vi "SSL Data Receiver.vi"(11 "SSL Data 2":refnum<vi>) -> (2 "SSL RefBox":T1, 3 "SSL Vision":T1)   [LabVIEW 2017]
uses:
  <extravilib>/ChannelInstances/Lossy Stream-a[.](u8)/)Channel.ctl
  Control/SSL Data Control.ctl
  Control/SSL UDP Address.ctl
  Control/File Player.ctl
  <extravilib>/ChannelInstances/Lossy Stream-a[.](u8)/Write With Abort.vi
  <extravilib>/ChannelInstances/Lossy Stream-a[.](u8)/Endpoint.vi
  <extravilib>/ChannelInstances/Stream-a[.](u8)/Instantiate.vi
  <extravilib>/ChannelInstances/Lossy Stream-a[.](u8)/Instantiate.vi
  <extravilib>/ChannelInstances/Lossy Stream-a[.](u8)/)Channel.vi
  <extravilib>/ChannelInstances/Lossy Stream-a[.](u8).lvlib
panel:
  in  "Boolean 2":refnum<vi>
  in  "Cluster in":refnum<vi>
  in  "RefBox UDP RX":refnum<vi>
  in  "SSL UDP RX":refnum<vi>
  out "error out":errorcluster
  out "error out 4":errorcluster
  out "error out":errorcluster
  # "UDP"
  # "LOG"
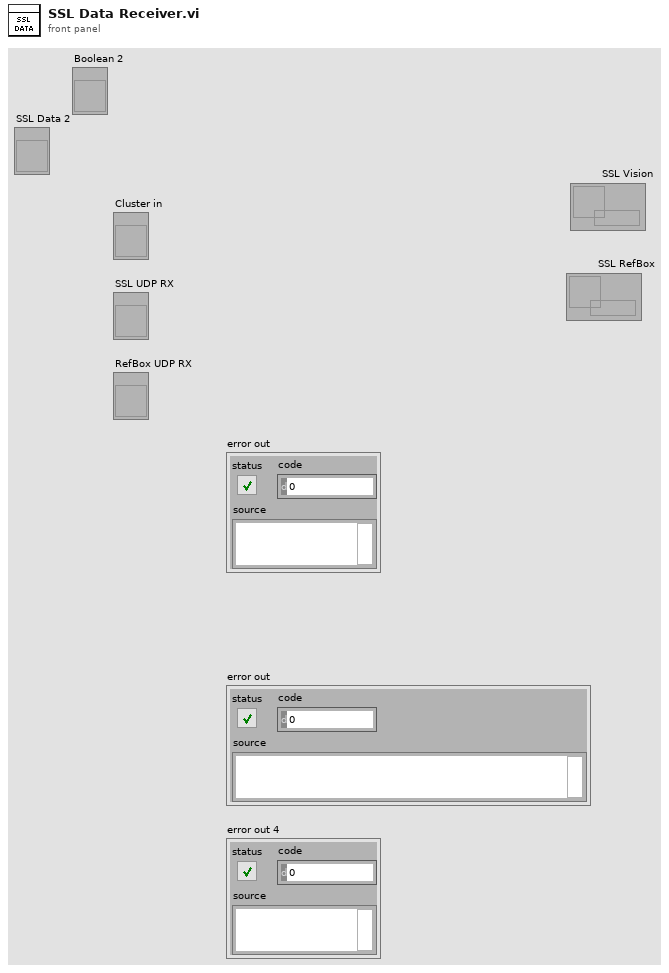
[diagram p1: front panel]
types:
  T1 = typedef "Lossy Stream-a[.](u8).lvlib/)Channel.ctl" = refnum<queue>
  T2 = typedef "Stream-a[.](u8).lvlib/)Channel.ctl" = refnum<queue>
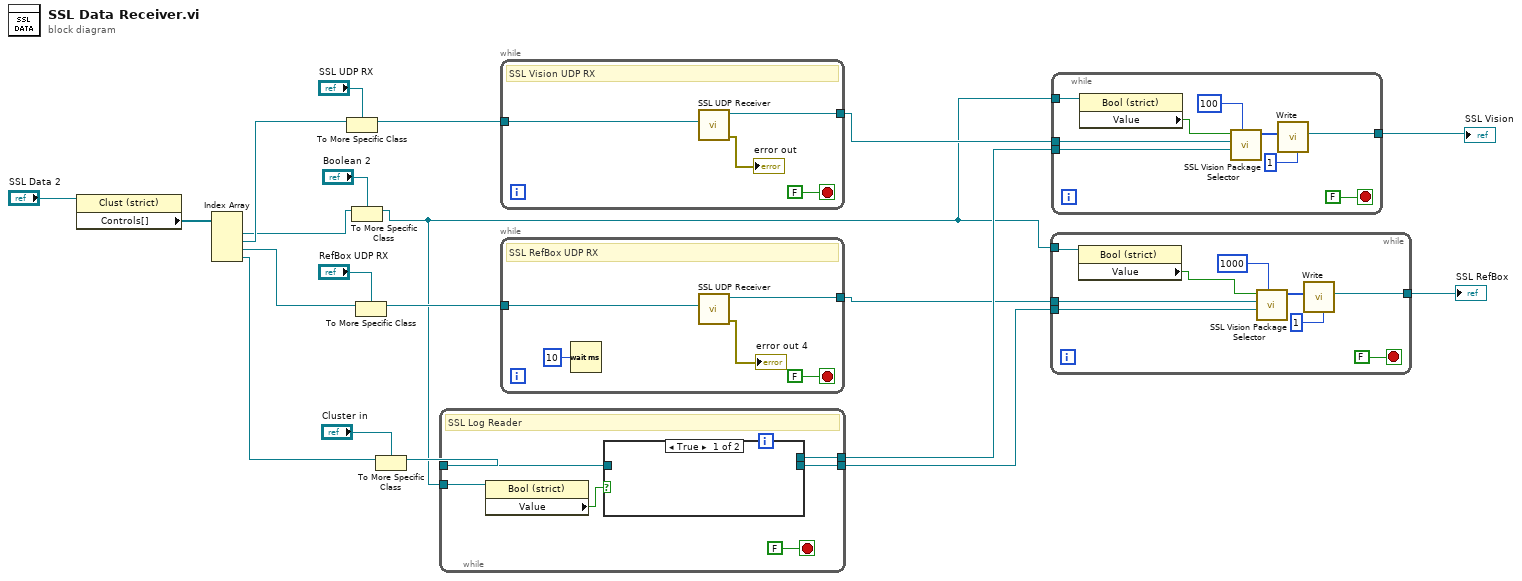
[diagram p0: block diagram]
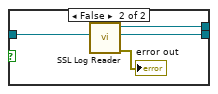
[diagram p2: hidden frame]
diagram:
  n1 = property on="Property Node" class="Clust (strict)"(reference="SSL Data 2") -> ("Controls[]"=w14:refnum<vi>[])  [unwired: 1 in, 2 out]
  n2 = Index Array(array=w14) -> (element #1=w2:refnum<vi>, element #2=w11:refnum<vi>, element #3=w8:refnum<vi>, element #4=w5:refnum<vi>)  [unwired: 4 in]
  n3 = To More Specific Class(target class="SSL UDP RX", reference=w11) -> (specific class reference=w12:refnum<vi>)  [unwired: 1 in, 1 out]
  n4 = To More Specific Class(target class="Boolean 2", reference=w2) -> (specific class reference=w1:refnum<vi>)  [unwired: 1 in, 1 out]
  n5 = To More Specific Class(target class="RefBox UDP RX", reference=w8) -> (specific class reference=w10:refnum<vi>)  [unwired: 1 in, 1 out]
  n6 = To More Specific Class(target class="Cluster in", reference=w5) -> (specific class reference=w7:refnum<vi>)  [unwired: 1 in, 1 out]
  n7 = while {
    tunnel: [w24] -> w17
    tunnel: [w25] -> w19
    tunnel: w7 -> [w23]
    tunnel: w1 -> [w22]
    stop <- FALSE stop-if-true
    # "SSL Log Reader"
    n8 = property class="Bool (strict)"(reference=w22) -> ("Value"=w21:bool)  [unwired: 1 in, 2 out]
    n9 = case shown="True" w21 {
      tunnel: [_ w29] -> w25
      tunnel: [_ w28] -> w24
      tunnel: w23 -> [_ w27]
      frame True {
      }
      frame False {
        n10 = call "SSL Log Reader.vi"("Cluster 2"=w27) -> ("error out"=→"error out":errorcluster, "channel 2"=w28:T2, "Channel out"=w29:T2)  [unwired: 7 in, 1 out]
      }
    }
  }
  n11 = while {
    tunnel: [w34] -> w20
    tunnel: w12 -> [w31]
    stop <- FALSE stop-if-true
    # "SSL Vision UDP RX"
    n12 = call "SSL UDP Receiver.vi"("SSL UDP Receiver 2"=w31) -> ("error out"=→"error out":errorcluster, "Channel out"=w34:T1)  [unwired: 9 in]
  }
  n13 = while {
    tunnel: [w37] -> w18
    tunnel: w10 -> [w36]
    stop <- FALSE stop-if-true
    # "SSL RefBox UDP RX"
    n14 = Wait (ms)(milliseconds to wait=u32 10) -> ()  [unwired: 1 out]
    n15 = call "SSL UDP Receiver.vi"("SSL UDP Receiver 2"=w36) -> ("error out"=→"error out 4":errorcluster, "Channel out"=w37:T1)  [unwired: 9 in]
  }
  n16 = while {
    tunnel: w18 -> [w48]
    tunnel: w17 -> [w47]
    tunnel: [w44] -> w16
    tunnel: w1 -> [w41]
    stop <- FALSE stop-if-true
    n17 = property class="Bool (strict)"(reference=w41) -> ("Value"=w42:bool)  [unwired: 1 in, 2 out]
    n18 = call "SSL Vision Package Selector.vi"("timeout in ms (-1)"=1000, "channel in"=w47, "Channel in"=w48, "Modo"=w42) -> ("element"=w45:u8[])  [unwired: 7 in]
    n19 = call <extravilib>:"Write.vi"("size (1)"=1, "element"=w45) -> ("channel"=w44:T1)  [unwired: 7 in, 2 out]
  }
  "SSL RefBox" <- w16
  n20 = while {
    tunnel: w20 -> [w57]
    tunnel: w19 -> [w56]
    tunnel: [w53] -> w15
    tunnel: w1 -> [w51]
    stop <- FALSE stop-if-true
    n21 = property class="Bool (strict)"(reference=w51) -> ("Value"=w50:bool)  [unwired: 1 in, 2 out]
    n22 = call "SSL Vision Package Selector.vi"("timeout in ms (-1)"=100, "channel in"=w56, "Channel in"=w57, "Modo"=w50) -> ("element"=w54:u8[])  [unwired: 7 in]
    n23 = call <extravilib>:"Write.vi"("size (1)"=1, "element"=w54) -> ("channel"=w53:T1)  [unwired: 7 in, 2 out]
  }
  "SSL Vision" <- w15
